vi "Sweep.vi"(8 "error in (no error)":errorcluster, 11 "Varian Continuous in":refnum<class "Varian Continuous.lvclass">) -> (0 "error out":errorcluster, 3 "Varian Continuous out":refnum<class "Varian Continuous.lvclass">)   [LabVIEW 2009, in "Varian Continuous.lvclass"]
uses:
  Varian Continuous.lvclass
  Instruments/Varian Magnet/Varian Magnet.lvclass
  Varian Continuous.lvclass/Varian Continuous.ctl
  Global/GPIB Numbers.vi
  <vilib>/DAQmx/create/channels.llb/DAQmx Create Channel (AO-Voltage-Basic).vi
  Instruments/Varian Magnet/Varian/Varian.lvlib
panel:
  out "Desired Field (T)":dbl[unit]
  out "Current field (T)":dbl[unit]
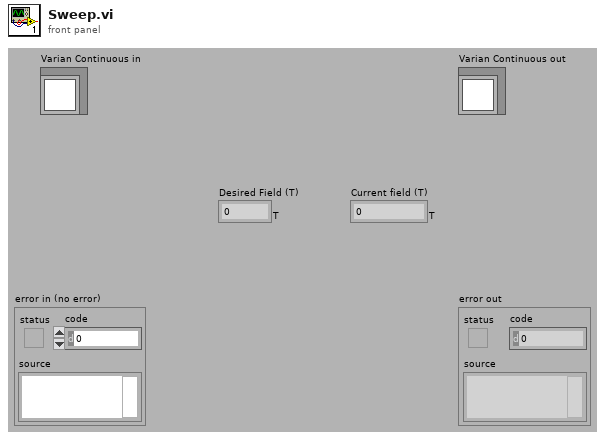
[diagram p1: front panel]
types:
  T1 = typedef "Scanner.lvclass/Range.ctl" = cluster{"xi":dbl, "xf":dbl, "dx":dbl, "Return to...?":bool, "Return to":dbl}
  T2 = typedef "GPIB Type Def.ctl" = cluster{"Name":string, "bus":dbl, "GPIB":dbl, "GPIB as string":string, "byte":i32, "VISA Resource Name":refnum<visa-resource-name>}
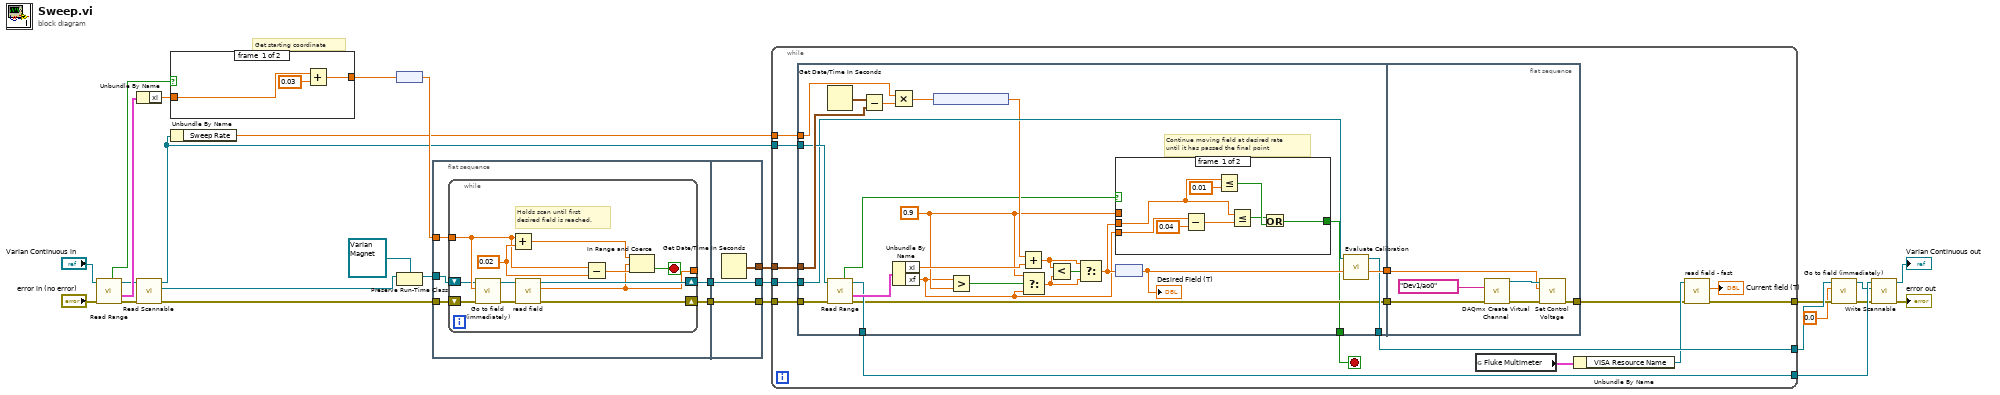
[diagram p0: block diagram]
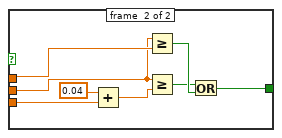
[diagram p2: hidden frame]
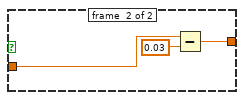
[diagram p3: hidden frame]
diagram:
  # "Get starting coordinate"
  n1 = call-dynamic "Read Range.vi"("error in (no error)"="error in (no error)", "Scanner.lvclass in"="Varian Continuous in") -> ("error out"=w20:errorcluster, "Range"=w25:T1, "Scanner.lvclass out"=w21:refnum<class "Varian Continuous.lvclass">, "Scanning Up?"=w26:bool)  [unwired: 4 in, 2 out]
  n2 = Unbundle By Name(w25) -> ("xi"=w24:dbl)
  n3 = call-dynamic "Read Scannable.vi"("error in (no error)"=w20, "Scanner.lvclass in"=w21) -> ("error out"=w19:errorcluster, "Scannable.lvclass"=w17:refnum<class "Scannable.lvclass">, "Scanner.lvclass out"=w7:refnum<class "Varian Continuous.lvclass">)  [unwired: 7 in]
  n4 = case shown="True" w26 {
    tunnel: w24 -> [w30 w33]
    tunnel: [w29 w32] -> w23
    frame #0 {
      n5 = Add(x=w30, y=0.03) -> (x+y=w29:dbl)
    }
    frame #1 {
      n6 = Subtract(x=w33, y=0.03) -> (x-y=w32:dbl)
    }
  }
  n7 = Unbundle By Name(w7) -> ("Sweep Rate"=w13:dbl[unit])
  n8 = node(w23) -> (w22:dbl[unit])
  n9 = Preserve Run-Time Class(object in=w17, 2:refnum<class "Varian Magnet.lvclass"> refnum ("Varian Magnet.lvclass")) -> (object out=w16:refnum<class "Varian Magnet.lvclass">)  [unwired: 1 in, 1 out]
  n10 = flat-sequence {
    tunnel: w22 -> [w39]
    tunnel: w19 -> [w38]
    tunnel: w16 -> [w37]
    tunnel: [w36] -> w15
    tunnel: [w35] -> w14
    tunnel: [w54] -> w11
    tunnel: w15 -> [w54]
    tunnel: [w53] -> w12
    tunnel: w14 -> [w53]
    tunnel: [w52] -> w6
    frame #0 {
      n11 = while {
        tunnel: [w42] -> _
        tunnel: w39 -> [w41]
        shift-right: [w44] -> w35
        shift-left: w38 -> [w45]
        shift-right: [w43] -> w36
        shift-left: w37 -> [w40]
        stop <- w46 stop-if-true
        w47 = dbl[unit] 0.02 ("y")
        # "Holds scan until first\ndesired field is reached."
        n12 = call "Go to field (immediately).vi"("error in"=w45, "Desired field (T)"=w41, "varian in"=w40) -> ("error out"=w51:errorcluster, "varian out"=w50:refnum<class "Varian Magnet.lvclass">)  [unwired: 7 in]
        n13 = Add(x=w41, y=w47) -> (x+y=w49:dbl[unit])
        n14 = call "read field.vi"("error in (no error)"=w51, "Varian Magnet.lvclass In"=w50) -> ("error out"=w44:errorcluster, "Field"=w42:dbl[unit], "Varian Magnet.lvclass Out"=w43:refnum<class "Varian Magnet.lvclass">)  [unwired: 7 in]
        n15 = Subtract(x=w41, y=w47) -> (x-y=w48:dbl[unit])
        n16 = In Range and Coerce(upper limit=w49, x=w42, lower limit=w48) -> (In Range?=w46:bool)  [unwired: 1 out]
      }
    }
    frame #1 {
      n17 = Get Date/Time In Seconds() -> (seconds since 1Jan1904=w52:timestamp)
    }
  }
  n18 = while {
    tunnel: w12 -> [w67]
    tunnel: w6 -> [w66]
    tunnel: w13 -> [w65]
    tunnel: [w64] -> w8
    tunnel: [w55] -> w4
    tunnel: w7 -> [w62]
    tunnel: w11 -> [w61]
    tunnel: [w60] -> w5
    stop <- w63 stop-if-true
    n19 = flat-sequence {
      tunnel: w67 -> [w94]
      tunnel: w66 -> [w92]
      tunnel: w65 -> [w80]
      tunnel: [w91] -> w69
      tunnel: [w78] -> w64
      tunnel: [w77] -> w68
      tunnel: [w89] -> w60
      tunnel: [w70] -> w63
      tunnel: w62 -> [w79]
      tunnel: w61 -> [w76]
      tunnel: w69 -> [w112]
      tunnel: [w111] -> w56
      tunnel: w68 -> [w113]
      frame #0 {
        w72 = 0.9
        # "Continue moving field at desired rate\nuntil it has passed the final point"
        n20 = Get Date/Time In Seconds() -> (seconds since 1Jan1904=w93:timestamp)
        n21 = call-dynamic "Read Range.vi"("error in (no error)"=w94, "Scanner.lvclass in"=w79) -> ("error out"=w77:errorcluster, "Range"=w83:T1, "Scanner.lvclass out"=w78:refnum<class "Varian Continuous.lvclass">, "Scanning Up?"=w74:bool)  [unwired: 4 in, 2 out]
        n22 = Subtract(x=w93, y=w92) -> (x-y=w82:dbl)
        n23 = Multiply(x=w80, y=w82) -> (x*y=w81:dbl[unit])
        n24 = Unbundle By Name(w83) -> ("xi"=w88:dbl, "xf"=w71:dbl)
        n25 = node(w81) -> (w75:dbl)
        n26 = Greater?(x=w71, y=w72) -> (0:w87:bool)
        n27 = Add(x=w75, y=w88) -> (x+y=w85:dbl)
        n28 = Select(t=w72, s=w87, f=w71) -> (s? t:f=w84:dbl)
        n29 = Less?(x=w85, y=w84) -> (x < y?=w86:bool)
        n30 = Select(t=w85, s=w86, f=w84) -> (s? t:f=w73:dbl)
        n31 = case shown="True" w74 {
          tunnel: w73 -> [w96 w104]
          tunnel: w72 -> [_ w109]
          tunnel: w71 -> [w98 w106]
          tunnel: [w99 w103] -> w70
          frame #0 {
            n32 = Subtract(x=w98, y=0.04) -> (x-y=w100:dbl)
            n33 = Less Or Equal?(x=w96, y=0.01) -> (x <= y?=w102:bool)
            n34 = Less Or Equal?(x=w96, y=w100) -> (x <= y?=w101:bool)
            n35 = Or(x=w101, y=w102) -> (x .or. y?=w99:bool)
          }
          frame #1 {
            n36 = Add(x=0.04, y=w106) -> (x+y=w105:dbl)
            n37 = Greater Or Equal?(x=w104, y=w109) -> (x >= y?=w110:bool)
            n38 = Greater Or Equal?(x=w104, y=w105) -> (x >= y?=w108:bool)
            n39 = Or(x=w108, y=w110) -> (x .or. y?=w103:bool)
          }
        }
        n40 = node(w73) -> (w90:dbl[unit])
        "Desired Field (T)" <- w90
        n41 = call "Evaluate Calibration.vi"("tesla"=w90, "varian in"=w76) -> ("control voltage"=w91:dbl, "varian out"=w89:refnum<class "Varian Magnet.lvclass">)  [unwired: 8 in]
      }
      frame #1 {
        n42 = call-poly <vilib>:"DAQmx Create Virtual Channel.vi"("physical channels"=tag "Dev1/ao0", "error in"=w113) -> ("task out"=w114:refnum<k21>, "error out"=w115:errorcluster)  [unwired: 7 in, 5 out]
        n43 = call "Set Control Voltage.vi"("error in"=w115, "Control Voltage"=w112, "task in"=w114) -> ("error out"=w111:errorcluster)  [unwired: 7 in, 1 out]
      }
    }
    n44 = global read "GPIB Numbers.vi" "Fluke Multimeter"() -> (w59:T2)
    n45 = Unbundle By Name(w59) -> ("VISA Resource Name"=w58:refnum<visa-resource-name>)
    n46 = call "read field - fast.vi"("error in (no error)"=w56, "VISA resource name"=w58) -> ("error out"=w55:errorcluster, "Current field (T)"=→"Current field (T)":dbl[unit])  [unwired: 7 in, 1 out]
  }
  n47 = call "Go to field (immediately).vi"("error in"=w4, "Desired field (T)"=dbl[unit] 0.0 ("y"), "varian in"=w5) -> ("error out"=w2:errorcluster, "varian out"=w1:refnum<class "Varian Magnet.lvclass">)  [unwired: 7 in]
  n48 = call-dynamic "Write Scannable.vi"("error in (no error)"=w2, "Scannable.lvclass"=w1, "Scanner.lvclass in"=w8) -> ("error out"=→"error out":errorcluster, "Scanner.lvclass out"=→"Varian Continuous out":refnum<class "Varian Continuous.lvclass">)  [unwired: 7 out]
